vi "Format for file.vi"(5 "Snapshot":T1={"Test Details"="", "Version"="test", "Date"=timestamp(0 s since 1904-01-01), "Selected Test"="", "Snapshot Number"=0, "Time"=timestamp(0 s since 1904-01-01), "Ibrake Setpoint"="", "RPM Setpoint"="", "Range Setpoint"="", "Step Height Setpoint"="", "Load Bank Setpoint"="", "Measurement Headers"="", "Measurements"="", "A"=0, "B"=0, "C"=0, "Raw Data"=[], "Available Tests"=enum."Manual", "Ibrake List"="", "RPM List"="", "Load Bank List"="", "Range List"="", "Step Height List"="", "FanMode Setpoint"=enum."Auto"} {"Time" format="%<%H:%M:%S>T"; "Date" format="%<%m/%d/%Y>T"}, 7 "Data Setup":refnum<vi>, 8 "error in (no error)":errorcluster, 9 "RPM":dbl, 10 "Torque":dbl, 11 "DAQmx Task Name":refnum<k21>) -> (0 "error out":errorcluster, 2 "Measurements":string, 3 "Headers and Measurements":string)   [LabVIEW 2017]
uses:
  Controls/Snapshot Typedef.ctl
  Controls/Available Tests.ctl
  Controls/FanMode.ctl
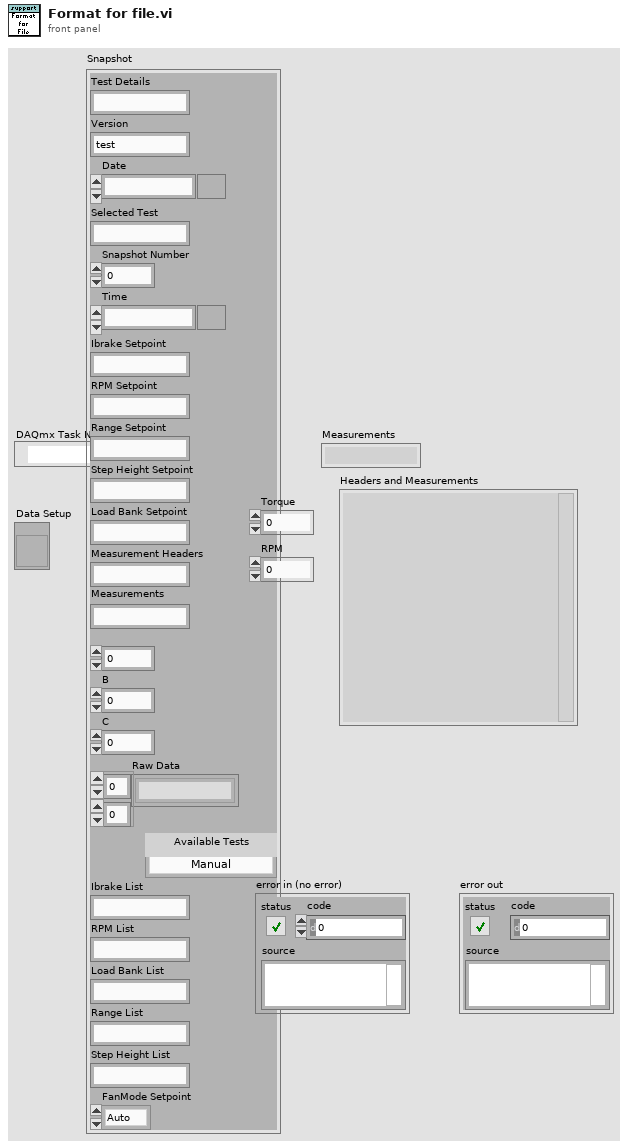
[diagram p1: front panel]
types:
  T1 = typedef "Snapshot Typedef.ctl" = cluster{"Test Details":string, "Version":string, "Date":timestamp, "Selected Test":string, "Snapshot Number":u16, "Time":timestamp, "Ibrake Setpoint":string, "RPM Setpoint":string, "Range Setpoint":string, "Step Height Setpoint":string, "Load Bank Setpoint":string, "Measurement Headers":string, "Measurements":string, "A":i32, "B":i32, "C":i32, "Raw Data":string[][], "Available Tests":T2, "Ibrake List":string, "RPM List":string, "Load Bank List":string, "Range List":string, "Step Height List":string, "FanMode Setpoint":T3}
  T2 = typedef "Available Tests.ctl" = enum16{"Manual", "EFX Brake Torque", "Generator Torque", "EFX Brake Thermal", "Generator Thermal", "Pulsed RPM", "AMT Brake Torque", "Bike Brake Torque", "AMT Brake Thermal", "Bike Brake Thermal"}
  T3 = typedef "FanMode.ctl" = enum16{"On", "Off", "Auto"}
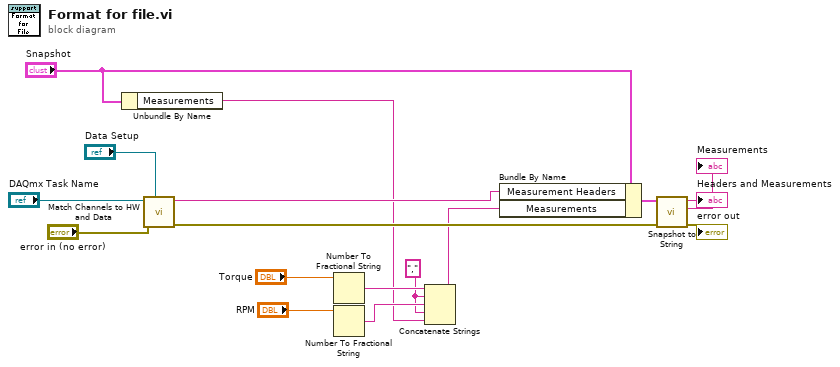
[diagram p0: block diagram]
diagram:
  w3 = ","
  n1 = Unbundle By Name("Snapshot") -> ("Measurements"=w1:string)
  n2 = call "Match Channels to HW and Data.vi"("Data Setup"="Data Setup", "error in (no error)"="error in (no error)", "DAQmx Task Name"="DAQmx Task Name") -> ("error IO"=w13:errorcluster, "Header"=w14:string)  [unwired: 6 in, 1 out]
  n3 = Number To Fractional String(number="Torque") -> (F-format string=w6:string)  [unwired: 3 in]
  n4 = Number To Fractional String(number="RPM") -> (F-format string=w5:string)  [unwired: 3 in]
  n5 = Concatenate Strings(w6, w3, w5, w3, w1) -> (w4:string)
  n6 = Bundle By Name(cluster="Snapshot", "Measurement Headers"=w14, "Measurements"=w4) -> (w15:T1)
  n7 = call "Snapshot to String.vi"("error in"=w13, "Snapshot"=w15) -> ("error out"=→"error out":errorcluster, "Measurements"=→"Measurements":string, "Headers and Measurements"=→"Headers and Measurements":string)  [unwired: 7 in]
